vi "Cam Attr.vi"() -> ()   [LabVIEW 2019]
uses:
  <vilib>/userDefined/High Color/IMAQdx.ctl
  <vilib>/vision/driver/IMAQdx.llb/IMAQdx Buffer Number Mode.ctl
  <vilib>/vision/driver/NI_Vision_Acquisition_Software.lvlib
  <resource>/objmgr/imaqdx.rc
panel:
  in  "Close":bool
  in  "Camera Name":T1="cam5"
  out "Image":T2(plugin-control)
  out "Temperature State":string
  out "Temperature Abs":dbl=61.0 format="%.2g"
  in  "Raw Gain":u32=1 max=360 step=1
  in  "Gain Auto":u32(ring) items=["OFF", "Once", "Continuous"]
  out "Acquired Frames per Second":u32=42
  in  "Frame Rate Abs":u32=100 min=1 max=100 step=1
  in  "Enable Acquisision FR":bool
  in  "Exposure Time Raw":u32=3000 min=34 max=10000000
  in  "Exposure Auto":u32(ring) items=["OFF", "Once", "Continuous"]
  in  "Frame Count":u32=1 max=255 step=1
  in  "Offset X":u32=8 max=4294966592 step=2
  in  "Width":u32=1920 min=2 max=1928 step=2
  in  "Offset Y":u32=8 max=16 step=2
  in  "Height":u32=1200 min=2 max=1208 step=2
  in  "Attributes":string(tree)
  out "Software name 2":string="Camera Setting"
  out "Software name":string="DSGS"
  out "time&date":string="2020/11/22"
  in  "error in":errorcluster
  out "error out":errorcluster
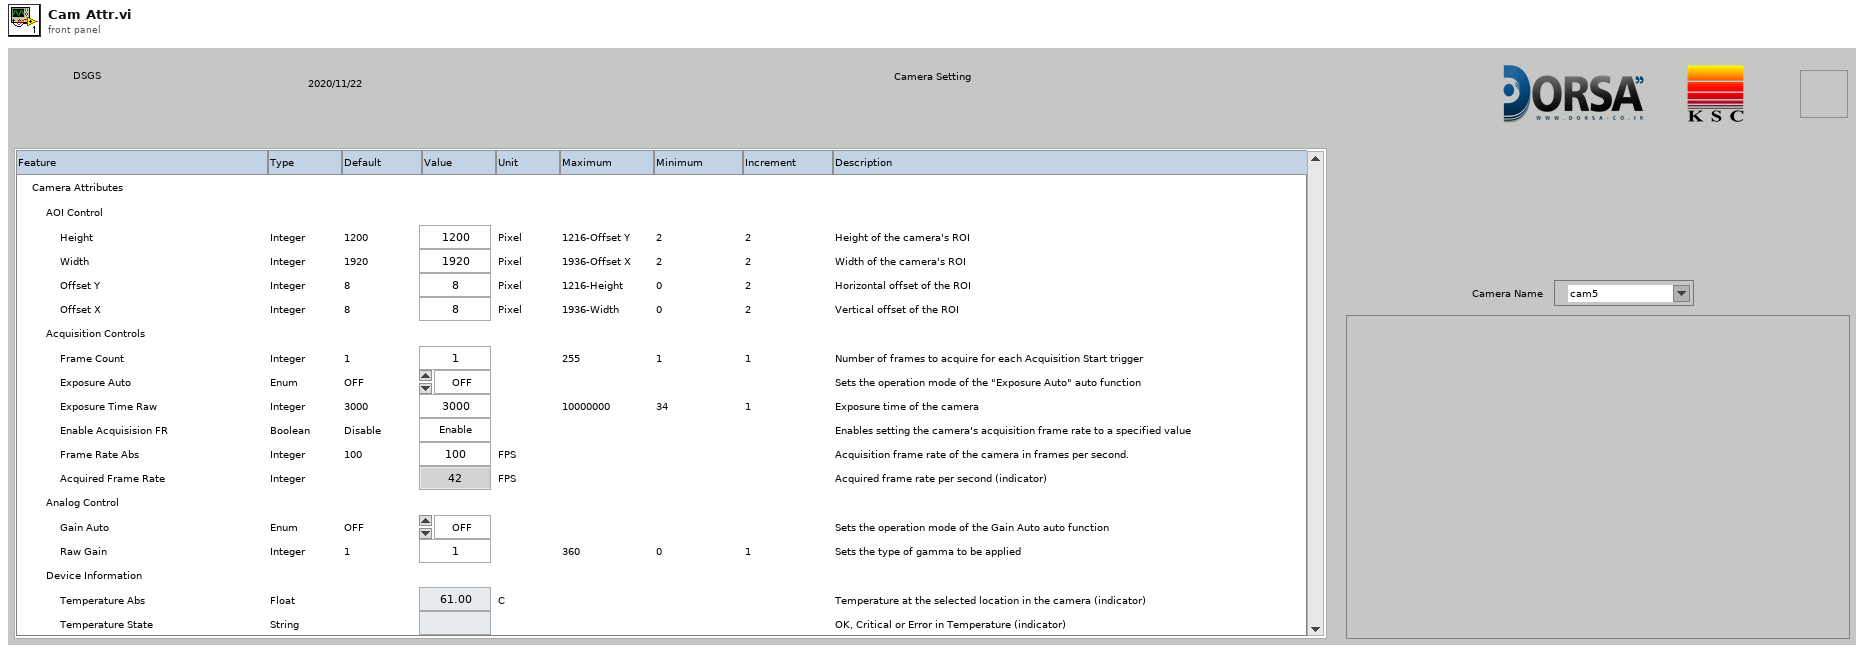
[diagram p1: front panel]
types:
  T1 = typedef "IMAQdx.ctl" = refnum<k21>
  T2 = typedef "IMAQ Image.ctl" = refnum<image>
  T3 = enum8{"Enabled", "Disabled", "Disabled and Grayed Out"}
  T4 = typedef "NI_Vision_Acquisition_Software.lvlib/IMAQdx Buffer Number Mode.ctl" = enum32{"Next", "Last", "Buffer Number", "Every", "Last New"}
  T5 = typedef "Image Type" = u32
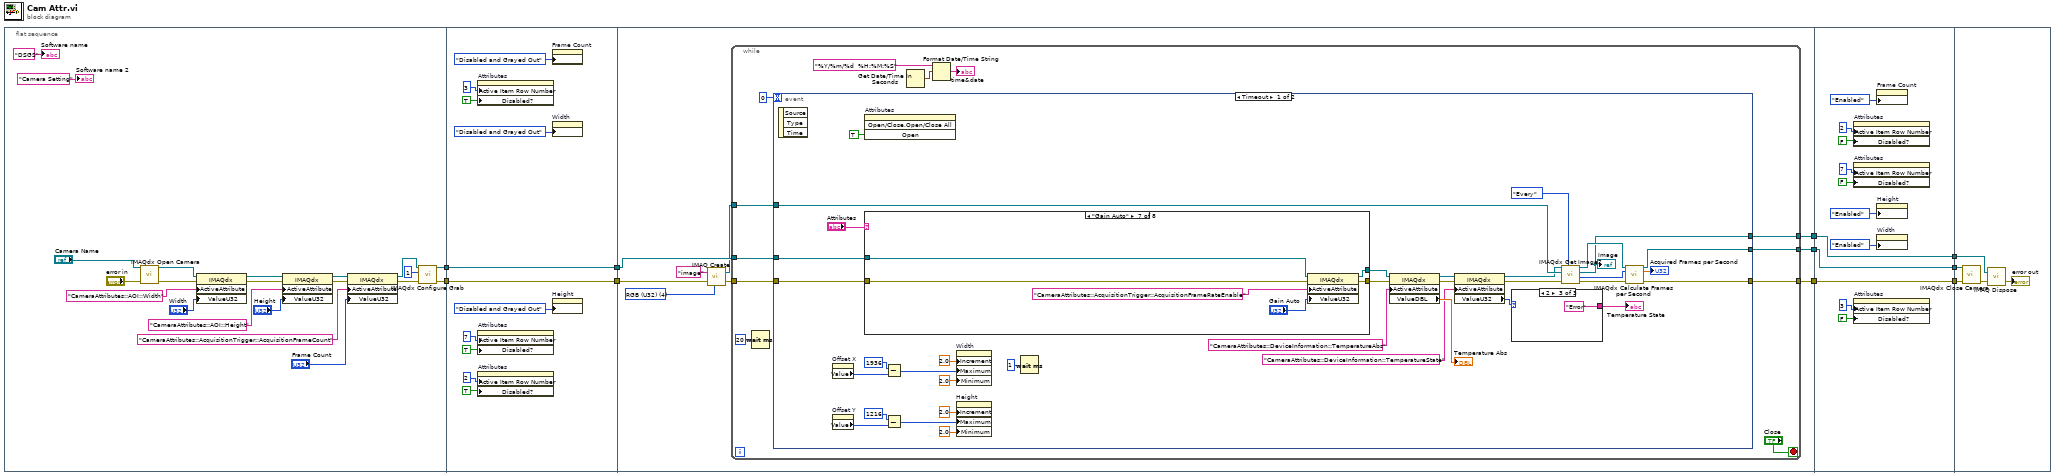
[diagram p0: block diagram]
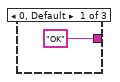
[diagram p2: hidden frame]
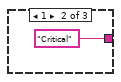
[diagram p3: hidden frame]
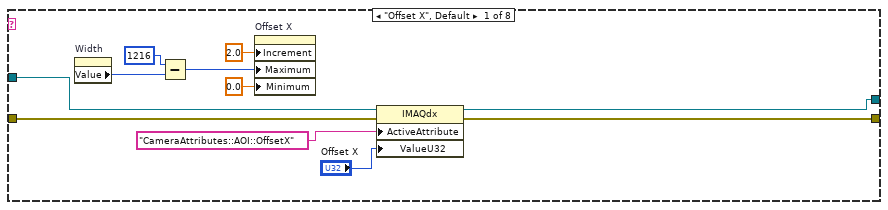
[diagram p4: hidden frame]
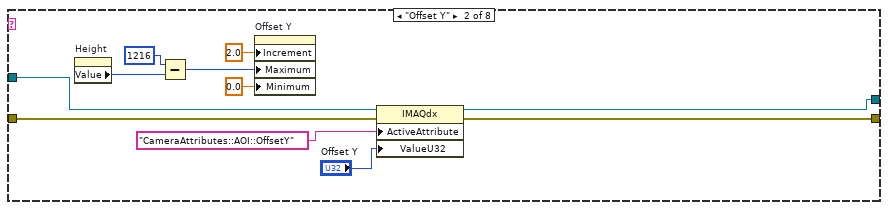
[diagram p5: hidden frame]
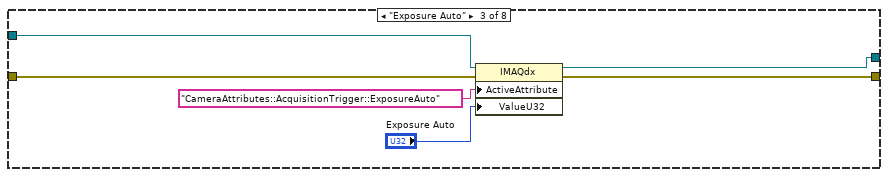
[diagram p6: hidden frame]
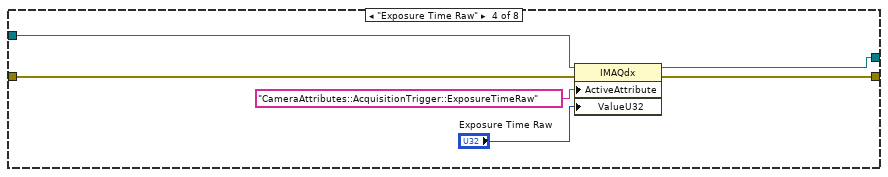
[diagram p7: hidden frame]
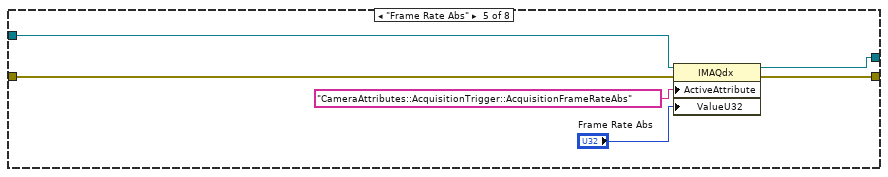
[diagram p8: hidden frame]
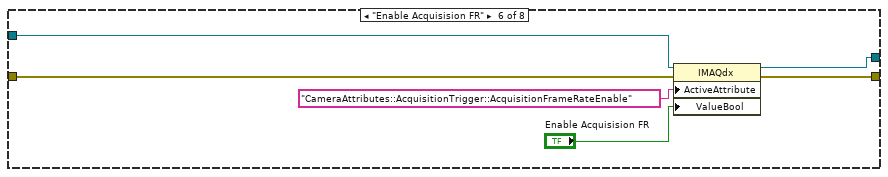
[diagram p9: hidden frame]
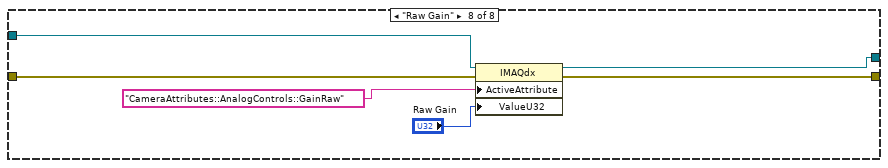
[diagram p10: hidden frame]
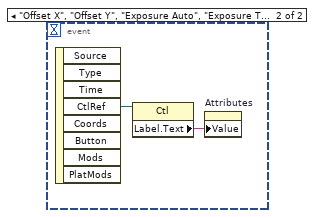
[diagram p11: hidden frame]
diagram:
  n1 = flat-sequence {
    tunnel: [w14] -> w10
    tunnel: [w13] -> w8
    tunnel: w10 -> [w42]
    tunnel: [w42] -> w9
    tunnel: w8 -> [w41]
    tunnel: [w41] -> w7
    tunnel: w9 -> [w48]
    tunnel: w7 -> [w49]
    tunnel: [w45] -> w6
    tunnel: [w44] -> w4
    tunnel: [w43] -> w2
    tunnel: w6 -> [w173]
    tunnel: [w173] -> w5
    tunnel: w4 -> [w172]
    tunnel: [w172] -> w3
    tunnel: w2 -> [w171]
    tunnel: [w171] -> w1
    tunnel: w5 -> [w175]
    tunnel: w3 -> [w174]
    tunnel: w1 -> [w177]
    frame #0 {
      n2 = call <vilib>:"IMAQdx Open Camera.vi"("error in"="error in", "Session In"="Camera Name") -> ("error out"=w27:errorcluster, "Session Out"=w18:T1)  [unwired: 8 in]
      n3 = property class="IMAQdx"(reference=w18, error in=w27, "ActiveAttribute"="CameraAttributes::AOI::Width", "ValueU32"="Width") -> (reference out=w24:T1, error out=w23:errorcluster)
      n4 = property class="IMAQdx"(reference=w24, error in=w23, "ActiveAttribute"="CameraAttributes::AOI::Height", "ValueU32"="Height") -> (reference out=w19:T1, error out=w20:errorcluster)
      n5 = property class="IMAQdx"(reference=w19, error in=w20, "ActiveAttribute"="CameraAttributes::AcquisitionTrigger::AcquisitionFrameCount", "ValueU32"="Frame Count") -> (reference out=w16:T1, error out=w15:errorcluster)
      n6 = call <vilib>:"IMAQdx Configure Grab.vi"("error in"=w15, "Number of Buffers"=u32 1, "Session In"=w16) -> ("error out"=w13:errorcluster, "Session Out"=w14:T1)  [unwired: 7 in]
      "Software name 2" <- "Camera Setting" ("Software name 2")
      "Software name" <- "DSGS" ("Software name")
    }
    frame #1 {
      n7 = property on="Attributes" class="Tree (strict)"("Active Item Row Number"=3 ("Active Item:Row Number"), "Disabled?"=TRUE ("Active Item:Disabled?")) -> ()  [unwired: 2 in, 2 out]
      n8 = property on="Attributes" class="Tree (strict)"("Active Item Row Number"=7 ("Active Item:Row Number"), "Disabled?"=TRUE ("Active Item:Disabled?")) -> ()  [unwired: 2 in, 2 out]
      n9 = property on="Attributes" class="Tree (strict)"("Active Item Row Number"=2 ("Active Item:Row Number"), "Disabled?"=TRUE ("Active Item:Disabled?")) -> ()  [unwired: 2 in, 2 out]
      n10 = property on="Frame Count" class="DigNum (strict)"("DisabledEnum"=T3."Disabled and Grayed Out" ("Disabled")) -> ()  [unwired: 2 in, 2 out]
      n11 = property on="Width" class="DigNum (strict)"("DisabledEnum"=T3."Disabled and Grayed Out" ("Disabled")) -> ()  [unwired: 2 in, 2 out]
      n12 = property on="Height" class="DigNum (strict)"("DisabledEnum"=T3."Disabled and Grayed Out" ("Disabled")) -> ()  [unwired: 2 in, 2 out]
    }
    frame #2 {
      w50 = T5 4 items=["Grayscale (U8)", "Grayscale (I16)", "Grayscale (SGL)", "Complex (CSG)", "RGB (U32)", "HSL (U32)", "RGB (U64)", "Grayscale (U16)"] ("Image Type")
      n13 = call "IMAQ Create"("Image Name"="image", "Image Type"=w50, "error in (no error)"=w49) -> ("New Image"=w46:T2, "error out"=w47:errorcluster)  [unwired: 2 in]
      n14 = while {
        tunnel: w48 -> [w63]
        tunnel: w47 -> [w62]
        tunnel: [w60] -> w45
        tunnel: [w59] -> w44
        tunnel: w46 -> [w61]
        tunnel: [w58] -> w43
        stop <- "Close" stop-if-true
        n15 = Wait (ms)(milliseconds to wait=u32 20) -> ()  [unwired: 1 out]
        n16 = event shown="[0] Timeout" {
          selector: _ -> [_ _]
          dyn-events: _ -> [_ _]
          timeout: 0 -> [_ _]
          tunnel: w63 -> [w96 _]
          tunnel: w62 -> [w95 _]
          tunnel: w61 -> [w83 _]
          tunnel: [w82 _] -> w60
          tunnel: [w81 _] -> w59
          tunnel: [w76 _] -> w58
          event Timeout {
            n17 = event-data() -> ()  [unwired: 1 in, 3 out]
            n18 = property on="Offset X" class="DigNum (strict)"() -> ("Value"=w91:u32)  [unwired: 2 in, 2 out]
            n19 = property on="Offset Y" class="DigNum (strict)"() -> ("Value"=w93:u32)  [unwired: 2 in, 2 out]
            n20 = invoke on="Attributes" class="Tree (strict)" method="Open/Close.Open/Close All"("Open"=TRUE ("Open?")) -> ()  [unwired: 3 in, 4 out]
            n21 = case shown="\"Gain Auto\"" "Attributes" {
              tunnel: w96 -> [w110 w121 w127 w131 w136 w144 w149 w157]
              tunnel: w95 -> [w109 w120 w126 w130 w137 w145 w148 w156]
              tunnel: [w112 w123 w129 w135 w141 w147 w151 w159] -> w67
              tunnel: [w111 w122 w128 w134 w140 w146 w150 w158] -> w66
              frame "Offset X", Default {
                n22 = property on="Width" class="DigNum (strict)"() -> ("Value"=w106:u32)  [unwired: 2 in, 2 out]
                n23 = Subtract(x=u32 1216, y=w106) -> (x-y=w105:u32)
                n24 = property on="Offset X" class="DigNum (strict)"("Increment"=2.0 ("Data Entry Limits:Increment"), "Maximum"=w105, "Minimum"=0.0 ("Data Entry Limits:Minimum")) -> ()  [unwired: 2 in, 2 out]
                n25 = property class="IMAQdx"(reference=w110, error in=w109, "ActiveAttribute"="CameraAttributes::AOI::OffsetX", "ValueU32"="Offset X") -> (reference out=w112:T1, error out=w111:errorcluster)
              }
              frame "Offset Y" {
                n26 = property on="Height" class="DigNum (strict)"() -> ("Value"=w116:u32)  [unwired: 2 in, 2 out]
                n27 = Subtract(x=u32 1216, y=w116) -> (x-y=w117:u32)
                n28 = property on="Offset Y" class="DigNum (strict)"("Increment"=2.0 ("Data Entry Limits:Increment"), "Maximum"=w117, "Minimum"=0.0 ("Data Entry Limits:Minimum")) -> ()  [unwired: 2 in, 2 out]
                n29 = property class="IMAQdx"(reference=w121, error in=w120, "ActiveAttribute"="CameraAttributes::AOI::OffsetY", "ValueU32"="Offset Y") -> (reference out=w123:T1, error out=w122:errorcluster)
              }
              frame "Exposure Auto" {
                n30 = property class="IMAQdx"(reference=w127, error in=w126, "ActiveAttribute"="CameraAttributes::AcquisitionTrigger::ExposureAuto", "ValueU32"="Exposure Auto") -> (reference out=w129:T1, error out=w128:errorcluster)
              }
              frame "Exposure Time Raw" {
                n31 = property class="IMAQdx"(reference=w131, error in=w130, "ActiveAttribute"="CameraAttributes::AcquisitionTrigger::ExposureTimeRaw", "ValueU32"="Exposure Time Raw") -> (reference out=w135:T1, error out=w134:errorcluster)
              }
              frame "Frame Rate Abs" {
                n32 = property class="IMAQdx"(reference=w136, error in=w137, "ActiveAttribute"="CameraAttributes::AcquisitionTrigger::AcquisitionFrameRateAbs", "ValueU32"="Frame Rate Abs") -> (reference out=w141:T1, error out=w140:errorcluster)
              }
              frame "Enable Acquisision FR" {
                n33 = property class="IMAQdx"(reference=w144, error in=w145, "ActiveAttribute"="CameraAttributes::AcquisitionTrigger::AcquisitionFrameRateEnable", "ValueBool"="Enable Acquisision FR") -> (reference out=w147:T1, error out=w146:errorcluster)
              }
              frame "Gain Auto" {
                n34 = property class="IMAQdx"(reference=w149, error in=w148, "ActiveAttribute"="CameraAttributes::AcquisitionTrigger::AcquisitionFrameRateEnable", "ValueU32"="Gain Auto") -> (reference out=w151:T1, error out=w150:errorcluster)
              }
              frame "Raw Gain" {
                n35 = property class="IMAQdx"(reference=w157, error in=w156, "ActiveAttribute"="CameraAttributes::AnalogControls::GainRaw", "ValueU32"="Raw Gain") -> (reference out=w159:T1, error out=w158:errorcluster)
              }
            }
            n36 = Subtract(x=u32 1936, y=w91) -> (x-y=w92:u32)
            n37 = Subtract(x=u32 1216, y=w93) -> (x-y=w94:u32)
            n38 = property on="Width" class="DigNum (strict)"("Increment"=2.0 ("Data Entry Limits:Increment"), "Maximum"=w92, "Minimum"=2.0 ("Data Entry Limits:Minimum")) -> ()  [unwired: 2 in, 2 out]
            n39 = property on="Height" class="DigNum (strict)"("Increment"=2.0 ("Data Entry Limits:Increment"), "Maximum"=w94, "Minimum"=2.0 ("Data Entry Limits:Minimum")) -> ()  [unwired: 2 in, 2 out]
            n40 = Wait (ms)(milliseconds to wait=u32 1) -> ()  [unwired: 1 out]
            n41 = property class="IMAQdx"(reference=w67, error in=w66, "ActiveAttribute"="CameraAttributes::DeviceInformation::TemperatureAbs") -> (reference out=w71:T1, error out=w72:errorcluster, "ValueDBL"=→"Temperature Abs":dbl)
            n42 = property class="IMAQdx"(reference=w71, error in=w72, "ActiveAttribute"="CameraAttributes::DeviceInformation::TemperatureState") -> (reference out=w64:T1, error out=w65:errorcluster, "ValueU32"=w73:u32)
            n43 = case shown="2" w73 {
              tunnel: ["OK" ("Temperature State") "Critical" ("Temperature State") "Error" ("Temperature State")] -> w74
              frame 0, Default {
              }
              frame 1 {
              }
              frame 2 {
              }
            }
            "Temperature State" <- w74
            n44 = call <vilib>:"IMAQdx Get Image2.vi"("Buffer Number Mode (Next)"=IMAQdx_Buffer_Number_Mode."Every", "error in"=w65, "Image In"=w83, "Session In"=w64) -> ("error out"=w78:errorcluster, "Buffer Number Out"=w80:u32, "Image Out"=w76:T2, "Session Out"=w79:T1)  [unwired: 4 in]
            "Image" <- w76
            n45 = call <vilib>:"IMAQdx Calculate Frames per Second.vi"("Session In"=w79, "Buffer Number"=w80, "error in (no error)"=w78) -> ("Session Out"=w82:T1, "Acquired Frames per Second"=→"Acquired Frames per Second":dbl, "error out"=w81:errorcluster)  [unwired: 6 in, 4 out]
          }
          event "Offset X", "Offset Y", "Exposure Auto", "Exposure Time Raw", "Enable Acquisision FR", "Frame Rate Abs", "Gain Auto", "Raw Gain": Mouse Down {
            n46 = event-data() -> ("CtlRef"=w161:refnum<vi>)  [unwired: 1 in, 7 out]
            n47 = property class="Ctl"(reference=w161) -> ("Label.Text"=w160:string)  [unwired: 1 in, 2 out]
            n48 = property on="Attributes" class="Tree (strict)"("Value"=w160) -> ()  [unwired: 2 in, 2 out]
          }
        }
        n49 = Get Date/Time In Seconds() -> (seconds since 1Jan1904=w54:timestamp)
        n50 = Format Date/Time String(time format string (%c)="%Y/%m/%d  %H:%M:%S", seconds (now)=w54) -> (date/time string=→"time&date":string)  [unwired: 1 in]
      }
    }
    frame #3 {
      n51 = property on="Attributes" class="Tree (strict)"("Active Item Row Number"=2 ("Active Item:Row Number"), "Disabled?"=FALSE ("Active Item:Disabled?")) -> ()  [unwired: 2 in, 2 out]
      n52 = property on="Attributes" class="Tree (strict)"("Active Item Row Number"=7 ("Active Item:Row Number"), "Disabled?"=FALSE ("Active Item:Disabled?")) -> ()  [unwired: 2 in, 2 out]
      n53 = property on="Attributes" class="Tree (strict)"("Active Item Row Number"=3 ("Active Item:Row Number"), "Disabled?"=FALSE ("Active Item:Disabled?")) -> ()  [unwired: 2 in, 2 out]
      n54 = property on="Frame Count" class="DigNum (strict)"("DisabledEnum"=T3."Enabled" ("Disabled")) -> ()  [unwired: 2 in, 2 out]
      n55 = property on="Height" class="DigNum (strict)"("DisabledEnum"=T3."Enabled" ("Disabled")) -> ()  [unwired: 2 in, 2 out]
      n56 = property on="Width" class="DigNum (strict)"("DisabledEnum"=T3."Enabled" ("Disabled")) -> ()  [unwired: 2 in, 2 out]
    }
    frame #4 {
      n57 = call <vilib>:"IMAQdx Close Camera.vi"("error in"=w174, "Session In"=w175) -> ("error out"=w176:errorcluster)  [unwired: 9 in]
      n58 = call "IMAQ Dispose"("Image"=w177, "error in (no error)"=w176) -> ("error out"=→"error out":errorcluster)  [unwired: 4 in]
    }
  }
